vi "Feedback Unit.vi"() -> ()   [LabVIEW 2020]
uses:
  Global Variables/Global Difficulty Level.vi
panel:
  out "NN Classification":dbl
  out "Level":i32
  out "Queue Error":errorcluster
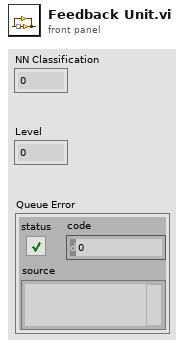
[diagram p1: front panel]
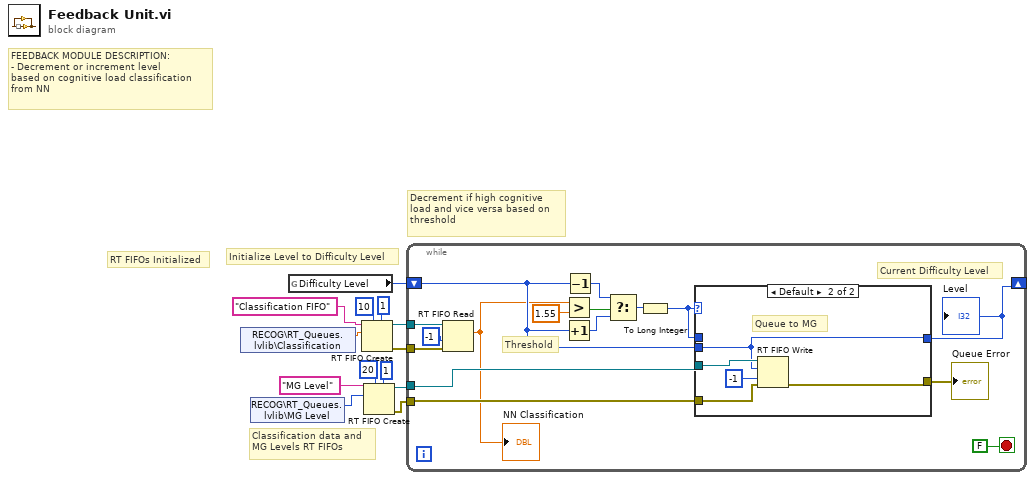
[diagram p0: block diagram]
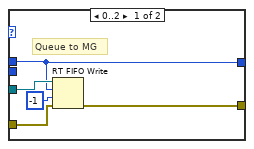
[diagram p2: hidden frame]
diagram:
  # "FEEDBACK MODULE DESCRIPTION: \n- Decrement or increment level \nbased on cognitive load classification \nfrom NN"
  # "Decrement if high cognitive \nload and vice versa based on \nthreshold"
  # "Classification data and \nMG Levels RT FIFOs"
  # "Initialize Level to Difficulty Level"
  # "RT FIFOs Initialized"
  n1 = shared-variable "RECOG\\RT_Queues.lvlib\\Classification"() -> (w13:dbl)  [unwired: 1 in, 1 out]
  n2 = shared-variable "RECOG\\RT_Queues.lvlib\\MG Level"() -> (w12:i32)  [unwired: 1 in, 1 out]
  n3 = global read "Global Difficulty Level.vi" "Difficulty Level"() -> (w1:u8)
  n4 = RT FIFO Create(0:"Classification FIFO" ("name (unnamed)"), 1:w13, 4:u32 10 ("size (10)"), 6:u32 1 ("elements in array (1)")) -> (8:w8:refnum<k33>, 11:w9:errorcluster)  [unwired: 4 in, 1 out]
  n5 = RT FIFO Create(0:"MG Level" ("FIFO"), 1:w12, 4:u32 20 ("size (10)"), 6:u32 1 ("elements in array (1)")) -> (8:w11:refnum<k33>, 11:w10:errorcluster)  [unwired: 4 in, 1 out]
  n6 = while {
    tunnel: w11 -> [w29]
    tunnel: w10 -> [w28]
    tunnel: w9 -> [w27]
    tunnel: w8 -> [w26]
    shift-right: [w24] -> _
    shift-left: w1 -> [w23]
    stop <- FALSE stop-if-true
    # "Current Difficulty Level"
    # "Threshold"
    n7 = RT FIFO Read(0:w26, 2:-1 ("timeout in ms (0)"), 3:w27) -> (9:w21:dbl)  [unwired: 1 in, 4 out]
    "NN Classification" <- w21
    n8 = Greater?(x=w21, y=1.55) -> (0:w20:bool)
    n9 = Increment(x=w23) -> (x+1=w18:i32)
    n10 = Decrement(x=w23) -> (x-1=w19:i32)
    n11 = Select(t=w19, s=w20, f=w18) -> (s? t:f=w17:i32)
    n12 = To Long Integer(number=w17) -> (32bit integer=w15:i32)
    n13 = case shown="Default" w15 {
      tunnel: w29 -> [w33 w38]
      tunnel: w28 -> [w32 w37]
      tunnel: w15 -> [w30 _]
      tunnel: [w31 w36] -> w14
      tunnel: [w30 w35] -> w24
      tunnel: w23 -> [_ w35]
      frame 0..2 {
        # "Queue to MG"
        n14 = RT FIFO Write(0:w33, 1:w30, 2:-1 ("timeout in ms (0)"), 3:w32) -> (11:w31:errorcluster)  [unwired: 1 in, 3 out]
      }
      frame Default {
        # "Queue to MG"
        n15 = RT FIFO Write(0:w38, 1:w35, 2:-1 ("timeout in ms (0)"), 3:w37) -> (11:w36:errorcluster)  [unwired: 1 in, 3 out]
      }
    }
    "Queue Error" <- w14
    "Level" <- w24
  }
